vi "PopulateRing.vi"(8 "error in":errorcluster) -> (0 "error out":errorcluster, 3 "Array":string[](array[string]))   [LabVIEW 2019, in "Scripts.lvclass"]
uses:
  Scripts.lvclass
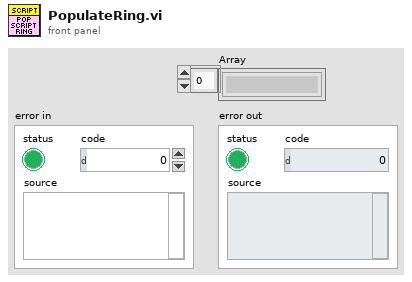
[diagram p1: front panel]
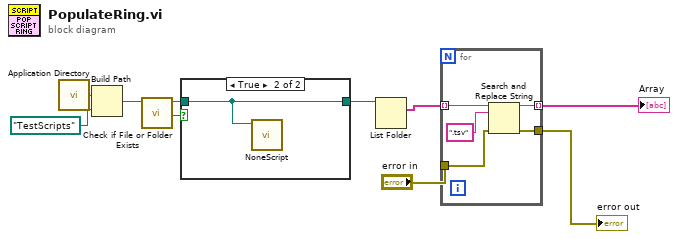
[diagram p0: block diagram]
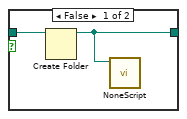
[diagram p2: hidden frame]
diagram:
  n1 = call <vilib>:"Application Directory.vi"() -> ("Application Directory"=w10:path)
  n2 = Build Path(base path=w10, name or relative path=path "TestScripts") -> (appended path=w4:path)
  n3 = call <vilib>:"Check if File or Folder Exists.vi"("path"=w4) -> ("file or folder exists?"=w5:bool, "dup path"=w1:path)  [unwired: 8 in, 1 out]
  n4 = case shown="True" w5 {
    tunnel: w1 -> [w12 w13]
    tunnel: [w11 w13] -> w3
    frame False {
      n5 = Create Folder(path (use dialog)=w12) -> (created path=w11:path)  [unwired: 2 in, 2 out]
      n6 = call "NoneScript.vi"("base path"=w11) -> ()  [unwired: 11 in]
    }
    frame True {
      n7 = call "NoneScript.vi"("base path"=w13) -> ()  [unwired: 11 in]
    }
  }
  n8 = List Folder(path=w3) -> (filenames=w2:string[])  [unwired: 3 in, 3 out]
  n9 = for {
    tunnel: [w17] -> w6 mode=indexing
    tunnel: [w16] -> w8
    tunnel: "error in" -> [w15]
    tunnel: w2 -> [w14] mode=indexing
    n10 = Search and Replace String(input string=w14, search string=".tsv", error in=w15) -> (result string=w17:string, error out=w16:errorcluster)  [unwired: 5 in, 2 out]
  }
  "error out" <- w8
  "Array" <- w6
